vi "GetBreakTag.vi"(8 "error in (no error)":errorcluster, 11 "LineBreak in":refnum<class "LineBreak.lvclass">) -> (0 "error out":errorcluster, 2 "BreakTag":string, 3 "LineBreak out":refnum<class "LineBreak.lvclass">)   [LabVIEW 2021, in "Markdown.lvlib" / "LineBreak.lvclass"]
uses:
  LineBreak.lvclass
  LineBreak.lvclass/LineBreak.ctl
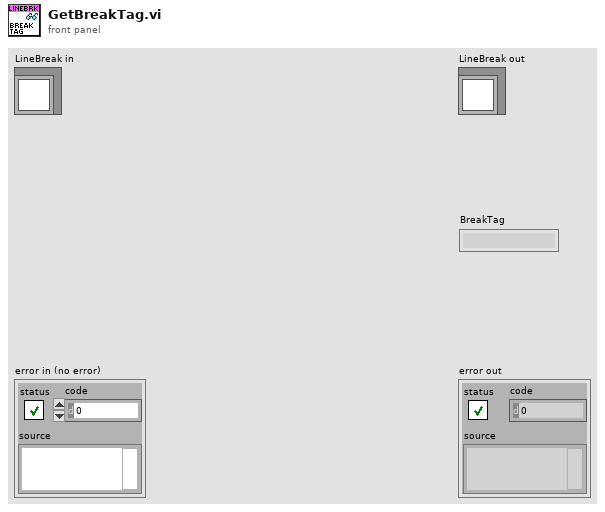
[diagram p1: front panel]
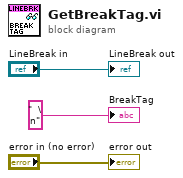
[diagram p0: block diagram]
diagram:
  "error out" <- "error in (no error)"
  "LineBreak out" <- "LineBreak in"
  "BreakTag" <- "  \n" ("BreakTag")
